vi "execute.vi"(8 "error in (no error)":errorcluster, 9 "data collection in":refnum<class "GenericComponent.lvclass">, 10 "imaging mode in":refnum<class "GenericComponent.lvclass">, 11 "AdapterCN091113ImagingModeToDataCollection in":refnum<class "AdapterCN091113ImagingModeToDataCollection.lvclass">) -> (0 "error out":errorcluster, 1 "data collection out":refnum<class "GenericComponent.lvclass">, 2 "imaging mode out":refnum<class "GenericComponent.lvclass">, 3 "AdapterCN091113ImagingModeToDataCollection out":refnum<class "AdapterCN091113ImagingModeToDataCollection.lvclass">)   [LabVIEW 2010, in "AdapterCN091113ImagingModeToDataCollection.lvclass"]
uses:
  AdapterCN091113ImagingModeToDataCollection.lvclass
  common/classes/GenericComponent/GenericComponent/GenericComponent.lvclass
  ImagingMode/ImagingModeDL100901FlexTrajectory/ImagingModeDL100901FlexTrajectory/ImagingModeDL100901FlexTrajectory.lvclass
  DataCollection/DataCollectionDL090215/DataCollectionDL090215/DataCollectionDL090215.lvclass
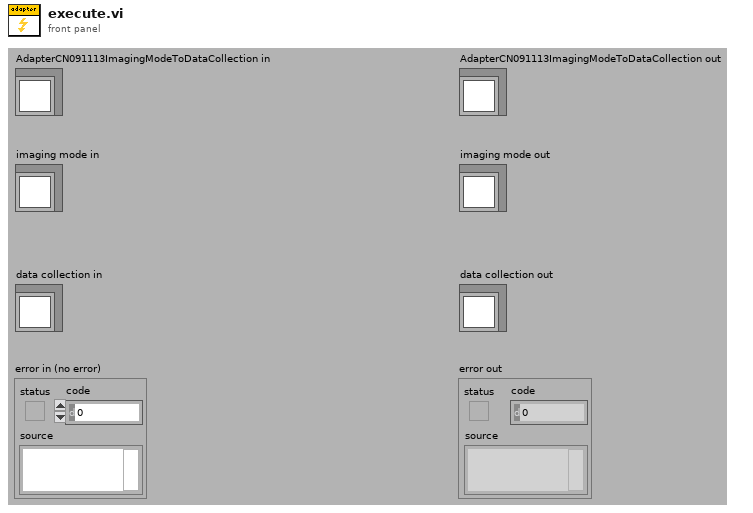
[diagram p1: front panel]
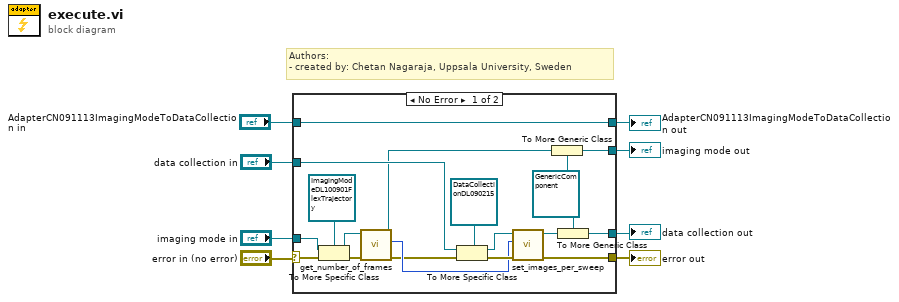
[diagram p0: block diagram]
diagram:
  # "Authors: \n- created by: Chetan Nagaraja, Uppsala University, Sweden"
  n1 = case shown="No Error" "error in (no error)" {
    selector: "error in (no error)" -> [w26 w29]
    tunnel: "imaging mode in" -> [w25 w27]
    tunnel: "data collection in" -> [w23 w28]
    tunnel: [w19 w27] -> w5
    tunnel: [w18 w29] -> w4
    tunnel: [w16 w28] -> w3
    tunnel: "AdapterCN091113ImagingModeToDataCollection in" -> [w15 w30]
    tunnel: [w15 w30] -> w1
    frame No Error {
      w20 = refnum<class "GenericComponent.lvclass"> refnum ("GenericComponent.lvclass")
      n2 = To More Specific Class(target class=refnum<class "ImagingModeDL100901FlexTrajectory.lvclass"> refnum ("ImagingModeDL100901FlexTrajectory.lvclass"), reference=w25, error in=w26) -> (specific class reference=w11:refnum<class "ImagingModeDL100901FlexTrajectory.lvclass">, error out=w12:errorcluster)
      n3 = call-dynamic "get_number_of_frames.vi"("error in (no error)"=w12, "ImagingModeDL100901FlexTrajectory in"=w11) -> ("error out"=w10:errorcluster, "number of frames"=w13:i32, "ImagingModeDL100901FlexTrajectory out"=w9:refnum<class "ImagingModeDL100901FlexTrajectory.lvclass">)  [unwired: 7 in]
      n4 = To More Specific Class(target class=refnum<class "DataCollectionDL090215.lvclass"> refnum ("DataCollectionDL090215.lvclass"), reference=w23, error in=w10) -> (specific class reference=w21:refnum<class "DataCollectionDL090215.lvclass">, error out=w22:errorcluster)
      n5 = call "set_images_per_sweep.vi"("error in (no error)"=w22, "images per sweep"=w13, "DataCollectionDL090215 in"=w21) -> ("error out"=w18:errorcluster, "DataCollectionDL090215 out"=w17:refnum<class "DataCollectionDL090215.lvclass">)  [unwired: 7 in]
      n6 = To More Generic Class(target class=w20, reference=w9) -> (generic class reference=w19:refnum<class "GenericComponent.lvclass">)
      n7 = To More Generic Class(target class=w20, reference=w17) -> (generic class reference=w16:refnum<class "GenericComponent.lvclass">)
    }
    frame Error {
    }
  }
  "error out" <- w4
  "AdapterCN091113ImagingModeToDataCollection out" <- w1
  "imaging mode out" <- w5
  "data collection out" <- w3
